vi "HS_AskVersion.vi"(8 "error in":errorcluster, 9 "Console In":string, 11 "VISA Refnum in":refnum<visa-resource-name>) -> (0 "error out":errorcluster, 1 "Console Out":string, 2 "Version":string, 3 "VISA Refnum out":refnum<visa-resource-name>)   [LabVIEW 2019]
panel:
  out "read buffer":string
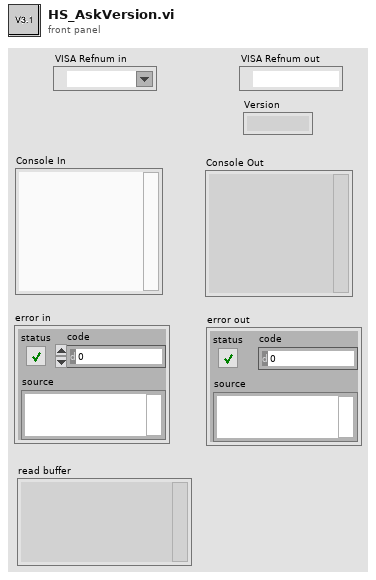
[diagram p1: front panel]
types:
  T1 = cluster{"Before":u8, "After":u8, "Send as 1 block?":bool}
  T2 = enum16{"big-endian, network order", "native, host order", "little-endian"}
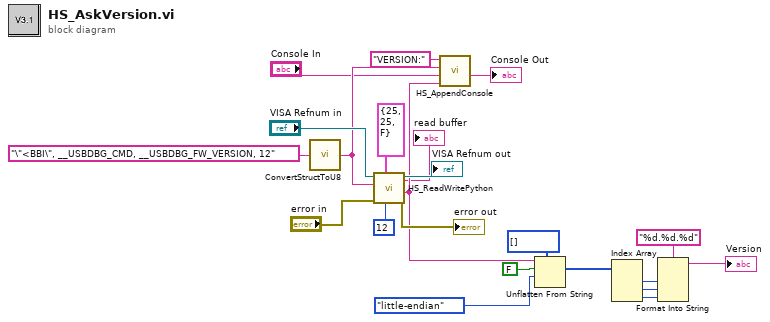
[diagram p0: block diagram]
diagram:
  n1 = call <userlib>:"ConvertStructToU8.vi"("struct"="\"<BBI\", __USBDBG_CMD, __USBDBG_FW_VERSION, 12" ("write buffer")) -> ("Binary"=w6:string)
  n2 = call <userlib>:"HS_ReadWritePython.vi"("Reply length"=12 ("Reply"), "Timeouts (ms)"=T1 {"Before"=25, "After"=25, "Send as 1 block?"=FALSE}, "error in"="error in", "Write"=w6, "VISA in"="VISA Refnum in") -> ("error out"=→"error out":errorcluster, "Console Out"=w4:string, "VISA out"=→"VISA Refnum out":refnum<visa-resource-name>, "read buffer"=→"read buffer":string)  [unwired: 1 in, 2 out]
  n3 = call <userlib>:"HS_AppendConsole.vi"("Reply"=w4, "Console in"="Console In", "Send"=w6, "Command"="VERSION:") -> ("Console Out"=→"Console Out":string)  [unwired: 7 in]
  n4 = Unflatten From String(type=i32[] [], binary string=w4, data includes array or string size? (T)=FALSE ("prepend array or string size? (T)"), byte order (0:big-endian, network order)=T2."little-endian") -> (value=w19:i32[])  [unwired: 1 in, 2 out]
  n5 = Index Array(array=w19) -> (element #1=w18:i32, element #2=w16:i32, element #3=w15:i32)  [unwired: 3 in]
  n6 = Format Into String(format string="%d.%d.%d", w18, w16, w15) -> (resulting string=→"Version":string)  [unwired: 2 in, 1 out]
